vi "CheckSHOT.vi"(8 "invader_in":T1={"output cluster"={"image type"=0, "image depth"=0, "image"=[], "mask"=[], "colors"=[], "Rectangle"={"left"=0, "top"=0, "right"=0, "bottom"=0}}, "direction"=enum."right", "shot_period"=0.0, "Speed"=10, "Bounds"={"Width"=0, "Height"=0}}, 11 "Array":T5(array[cluster])) -> (3 "SHOT":bool)   [LabVIEW 2019]
uses:
  invader.ctl
  <vilib>/picture/picture.llb/imagedata.ctl
  move_dir_lr.ctl
  <vilib>/Utility/miscctls.llb/LVBoundsTypeDef.ctl
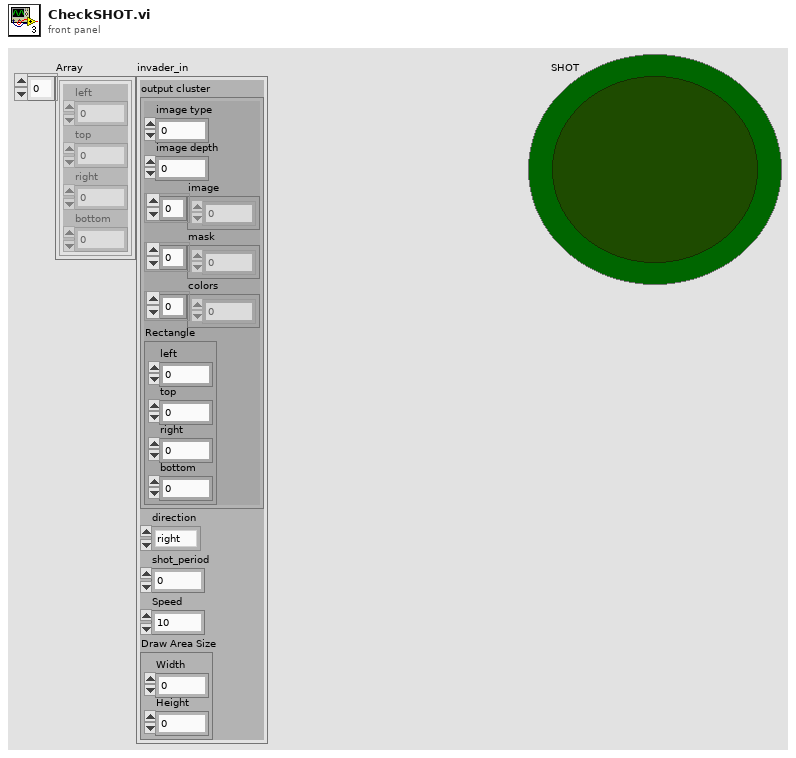
[diagram p1: front panel]
types:
  T1 = typedef "invader.ctl" = cluster{"output cluster":T2, "direction":T3, "shot_period":dbl, "Speed":i16, "Bounds":T4}
  T2 = typedef "imagedata.ctl" = cluster{"image type":i32, "image depth":i32, "image":u8[], "mask":u8[], "colors":u32[], "Rectangle":cluster{"left":i16, "top":i16, "right":i16, "bottom":i16}}
  T3 = typedef "move_dir_lr.ctl" = enum16{"right", "left"}
  T4 = typedef "LVBoundsTypeDef.ctl" = cluster{"Width":u32, "Height":u32}
  T5 = cluster{"left":i16, "top":i16, "right":i16, "bottom":i16}[]
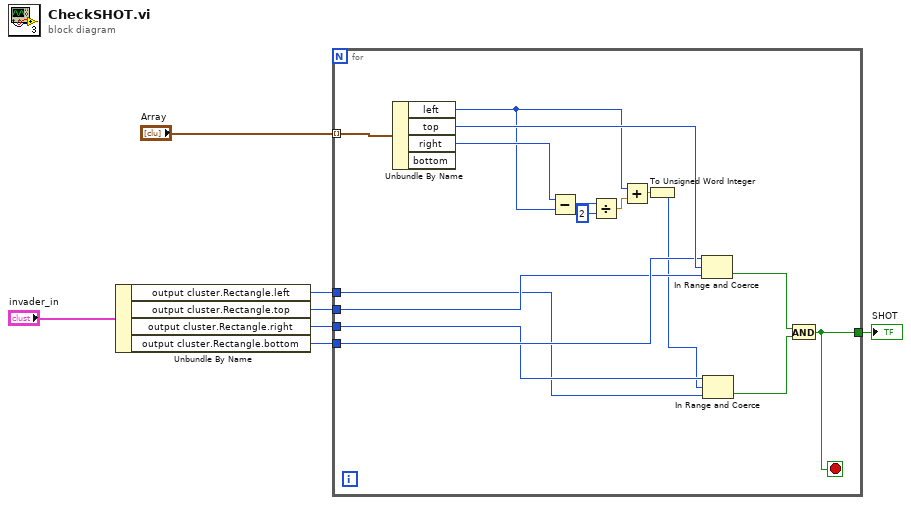
[diagram p0: block diagram]
diagram:
  n1 = Unbundle By Name("invader_in") -> ("output cluster.Rectangle.left"=w1:i16, "output cluster.Rectangle.top"=w5:i16, "output cluster.Rectangle.right"=w2:i16, "output cluster.Rectangle.bottom"=w4:i16)
  n2 = for {
    tunnel: "Array" -> [w23] mode=indexing
    tunnel: w1 -> [w15]
    tunnel: w5 -> [w20]
    tunnel: w2 -> [w19]
    tunnel: w4 -> [w21]
    tunnel: [w16] -> w3
    stop <- w16 stop-if-true
    n3 = Unbundle By Name(w23) -> ("left"=w9:i16, "top"=w22:i16, "right"=w10:i16)  [unwired: 1 out]
    n4 = Subtract(x=w10, y=w9) -> (x-y=w12:i16)
    n5 = Divide(x=w12, y=i16 2) -> (x/y=w13:dbl)
    n6 = Add(x=w9, y=w13) -> (x+y=w14:dbl)
    n7 = To Unsigned Word Integer(number=w14) -> (unsigned 16bit integer=w8:u16)
    n8 = In Range and Coerce(upper limit=w21, x=w22, lower limit=w20) -> (In Range?=w18:bool)  [unwired: 1 out]
    n9 = In Range and Coerce(upper limit=w19, x=w8, lower limit=w15) -> (In Range?=w17:bool)  [unwired: 1 out]
    n10 = And(x=w18, y=w17) -> (x .and. y?=w16:bool)
  }
  "SHOT" <- w3
